vi "CNTRLR - Fire Command.vi"(8 "error in (no error)":errorcluster, 9 "Data":variant, 10 "CMD":T1, 11 "View Model":T2) -> (0 "error out":errorcluster)   [LabVIEW 2017]
doc: "Generates User Event = Command to Car Wash CNTRLR with parameters (Data)."
uses:
  View Model/Controls/View Model.ctl
  View Model/Controls/Shared Model.ctl
  Error Handler/Controls/Error Model.ctl
  Error Handler/Controls/Error Message.ctl
  Error Handler/Controls/Error Level.ctl
  Configuration/Controls/Database Model.ctl
  Configuration/Controls/Database Message.ctl
  Configuration/Controls/Database Command.ctl
  Configuration/Controls/Database Overhead.ctl
  Configuration/Controls/Database Status.ctl
  Configuration/Controls/Database Record.ctl
  Controls/CNTRLR - Model.ctl
  Controls/CNTRLR - Message.ctl
  Controls/CNTRLR - Command.ctl
  Controls/CNTRLR - Overhead.ctl
  Controls/CNTRLR - Position.ctl
  Controls/CNTRLR - State.ctl
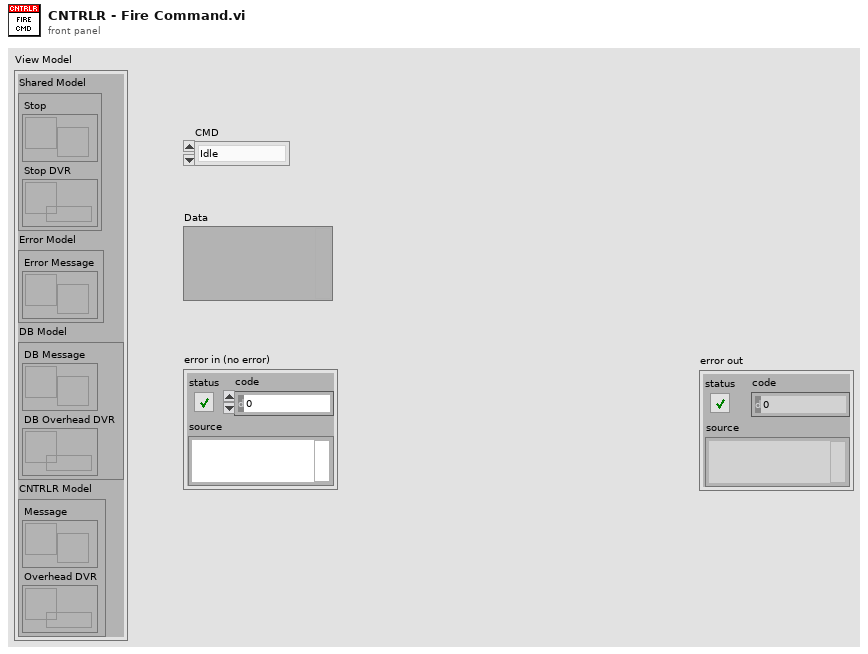
[diagram p1: front panel]
types:
  T1 = typedef "CNTRLR - Command.ctl" = enum16{"Idle", "Start Car Wash", "Error"}
  T2 = typedef "View Model.ctl" = cluster{"Shared Model":T3, "Error Model":T4, "DB Model":T5, "CNTRLR Model":T6}
  T3 = typedef "Shared Model.ctl" = cluster{"Stop":refnum<user-event>, "Stop DVR":refnum<data-value>}
  T4 = typedef "Error Model.ctl" = cluster{"Error Message":refnum<user-event>}
  T5 = typedef "Database Model.ctl" = cluster{"DB Message":refnum<user-event>, "DB Overhead DVR":refnum<data-value>}
  T6 = typedef "CNTRLR - Model.ctl" = cluster{"Message":refnum<user-event>, "Overhead DVR":refnum<data-value>}
  T7 = typedef "CNTRLR - Message.ctl" = cluster{"CMD":T1, "Data":variant}
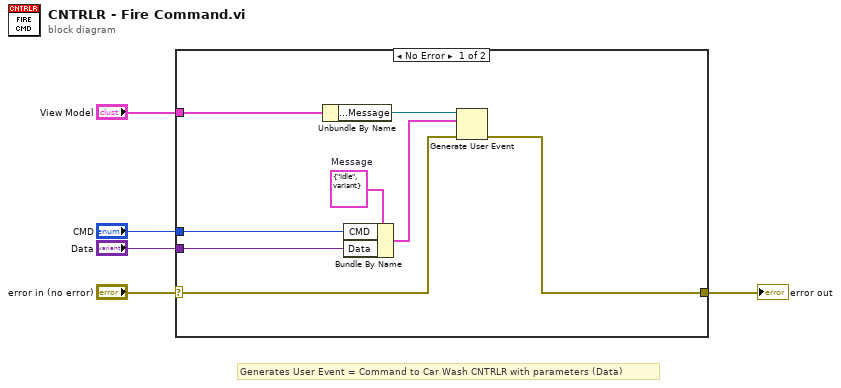
[diagram p0: block diagram]
diagram:
  # "Generates User Event = Command to Car Wash CNTRLR with parameters (Data)"
  n1 = case shown="No Error" "error in (no error)" {
    selector: "error in (no error)" -> [w7 w14]
    tunnel: [w6 w14] -> w4
    tunnel: "View Model" -> [w13 _]
    tunnel: "Data" -> [w10 _]
    tunnel: "CMD" -> [w9 _]
    frame No Error {
      w11 = T7 {"CMD"=enum."Idle", "Data"=variant}  # Message
      n2 = Unbundle By Name(w13) -> ("CNTRLR Model.Message"=w12:refnum<user-event>)
      n3 = Bundle By Name(cluster=w11, "CMD"=w9, "Data"=w10) -> (w8:T7)
      n4 = Generate User Event(user event=w12, event data cluster=w8, error in=w7) -> (error out=w6:errorcluster)  [unwired: 1 in, 1 out]
    }
    frame Error {
    }
  }
  "error out" <- w4
